vi "ex_confReadSampleFile.vi"(2 "First Row is Channel Names":bool, 3 "Generic Params":T1, 4 "Expanded path":path) -> (0 "error out":errorcluster, 1 "Sample Data":string[][](array[string]))   [LabVIEW 2020]
uses:
  <vilib>/express/express input/ExFileReadBlock.llb/ex_ReadFileGenericParams.ctl
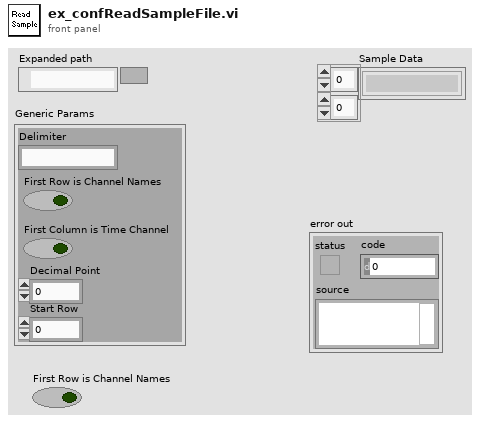
[diagram p1: front panel]
types:
  T1 = typedef "ex_ReadFileGenericParams.ctl" = cluster{"Delimiter":string, "First Row is Channel Names":bool, "First Column is Time Channel":bool, "Decimal Point":i32, "Start Row":i32}
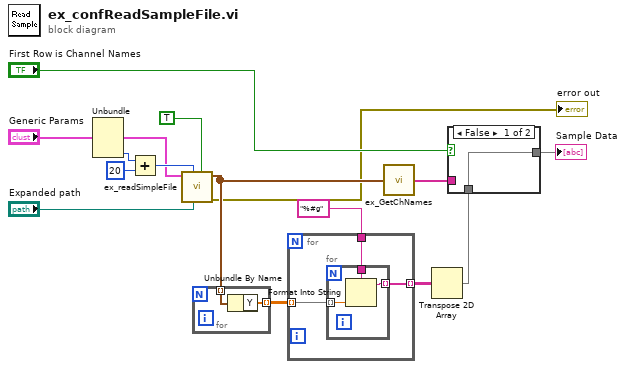
[diagram p0: block diagram]
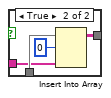
[diagram p2: hidden frame]
diagram:
  n1 = Unbundle("Generic Params") -> ("Start Row"=w2:i32)  [unwired: 4 out]
  n2 = Add(x=w2, y=20 ("number of lines (all:-1)")) -> (x+y=w4:i32)
  n3 = call <vilib>:"ex_readSimpleFile.vi"("first time"=TRUE, "Path"="Expanded path", "number of lines (all:-1)"=w4, "Generic Params"="Generic Params") -> ("error out"=→"error out":errorcluster, "Signals"=w10:waveform(dbl)[])  [unwired: 3 in, 3 out]
  n4 = for {
    tunnel: w10 -> [w17] mode=indexing
    tunnel: [w16] -> w8 mode=indexing
    n5 = Unbundle By Name(w17) -> ("Y"=w16:dbl[])
  }
  n6 = for {
    tunnel: "%#g" ("format string") -> [w20]
    tunnel: w8 -> [w19] mode=indexing
    tunnel: [w18] -> w9 mode=indexing
    n7 = for {
      tunnel: w20 -> [w23]
      tunnel: w19 -> [w22] mode=indexing
      tunnel: [w21] -> w18 mode=indexing
      n8 = Format Into String(format string=w23, w22) -> (resulting string=w21:string)  [unwired: 2 in, 1 out]
    }
  }
  n9 = call <vilib>:"ex_GetChNames.vi"("Signals"=w10) -> ("Channel Names"=w12:string[])
  n10 = Transpose 2D Array(2D array=w9) -> (transposed array=w11:string[][])
  n11 = case shown="False" "First Row is Channel Names" {
    tunnel: w11 -> [w24 w28]
    tunnel: w12 -> [_ w27]
    tunnel: [w24 w26] -> w14
    frame False {
    }
    frame True {
      n12 = Insert Into Array(array=w28, index (row)=0, new element=w27) -> (w26:string[][])  [unwired: 1 in]
    }
  }
  "Sample Data" <- w14
